vi "Read BM Messages.vi"(0 "Bus Config Info":T1, 11 "error in (no error)":errorcluster) -> (4 "VP BM Messages Read":T3[](array[typedef]) {"Data Word array" format="%x"}, 8 "Data Available":bool, 15 "error out":errorcluster)   [LabVIEW 2013, in "AIT 1553 Custom Device.lvlib"]
uses:
  AIT 1553 Custom Device.lvlib
  RT Controls/VP_BM Message.ctl
  RT Controls/AIT 1553 - Board Config Info.ctl
  RT Controls/AIT 1553 - Hardware Type.ctl
  <instrlib>/AIT 1553/AIT 1553.lvlib
  <userlib>/MIL-STD-1553/Owl1553.lvlib
  <vilib>/NI Veristand/Custom Device Tools/Custom Device Utility Library/Custom Device Utility Library.lvlib
  <vilib>/NI Veristand/Custom Device Tools/Custom Device Utility Library/RT Debug String Color Spec.ctl
panel:
  out "BM Read Exec Time":u32
  out "words read out":i32
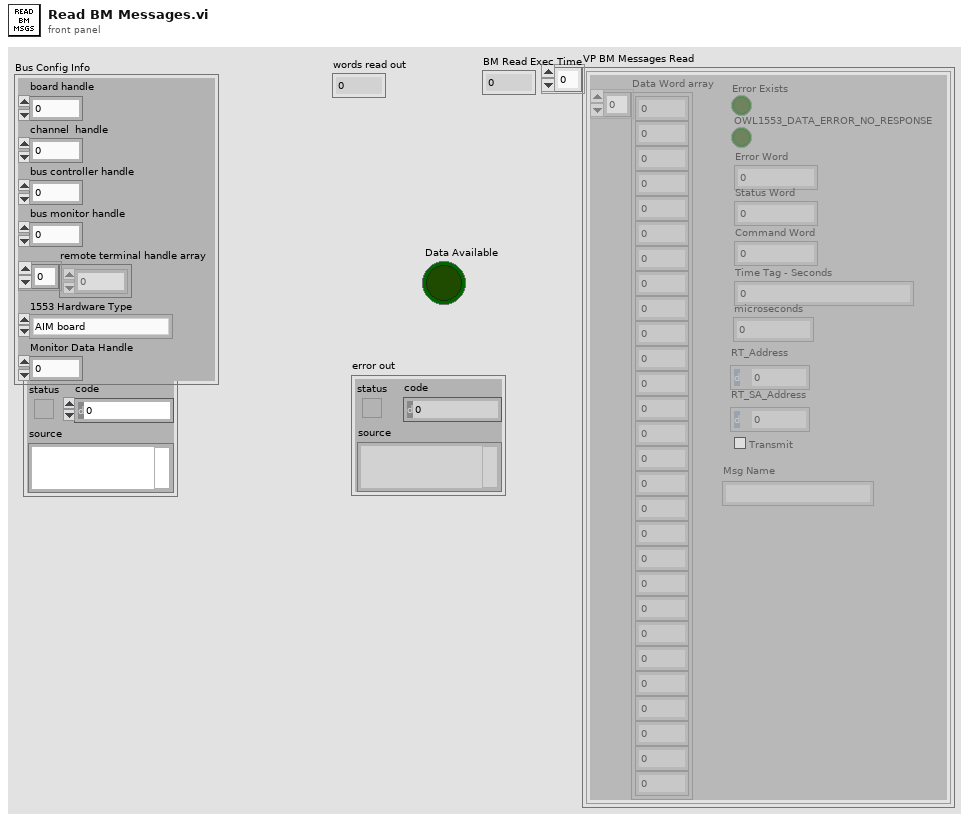
[diagram p1: front panel]
types:
  T1 = typedef "AIT 1553 Custom Device.lvlib/AIT 1553 - Board Config Info.ctl" = cluster{"board handle":u32, "channel  handle":u32, "bus controller handle":u32, "bus monitor handle":u32, "remote terminal handle array":u32[], "1553 Hardware Type":T2, "Monitor Data Handle":u32}
  T2 = typedef "AIT 1553 Custom Device.lvlib/AIT 1553 - Hardware Type.ctl" = enum16{"AIM board", "AIT Board"}
  T3 = typedef "AIT 1553 Custom Device.lvlib/VP_BM Message.ctl" = cluster{"Data Word array":u16[], "Error Exists":bool, "OWL1553_DATA_ERROR_NO_RESPONSE":bool, "Error Word":u32, "Status Word":u16, "Command Word":u16, "Time Tag - Seconds":u32, "microseconds":u32, "RT_Address":u8, "RT_SA_Address":u8, "Transmit":bool, "Msg Name":string}
  T4 = typedef "Custom Device Utility Library.lvlib/RT Debug String Color Spec.ctl" = u16
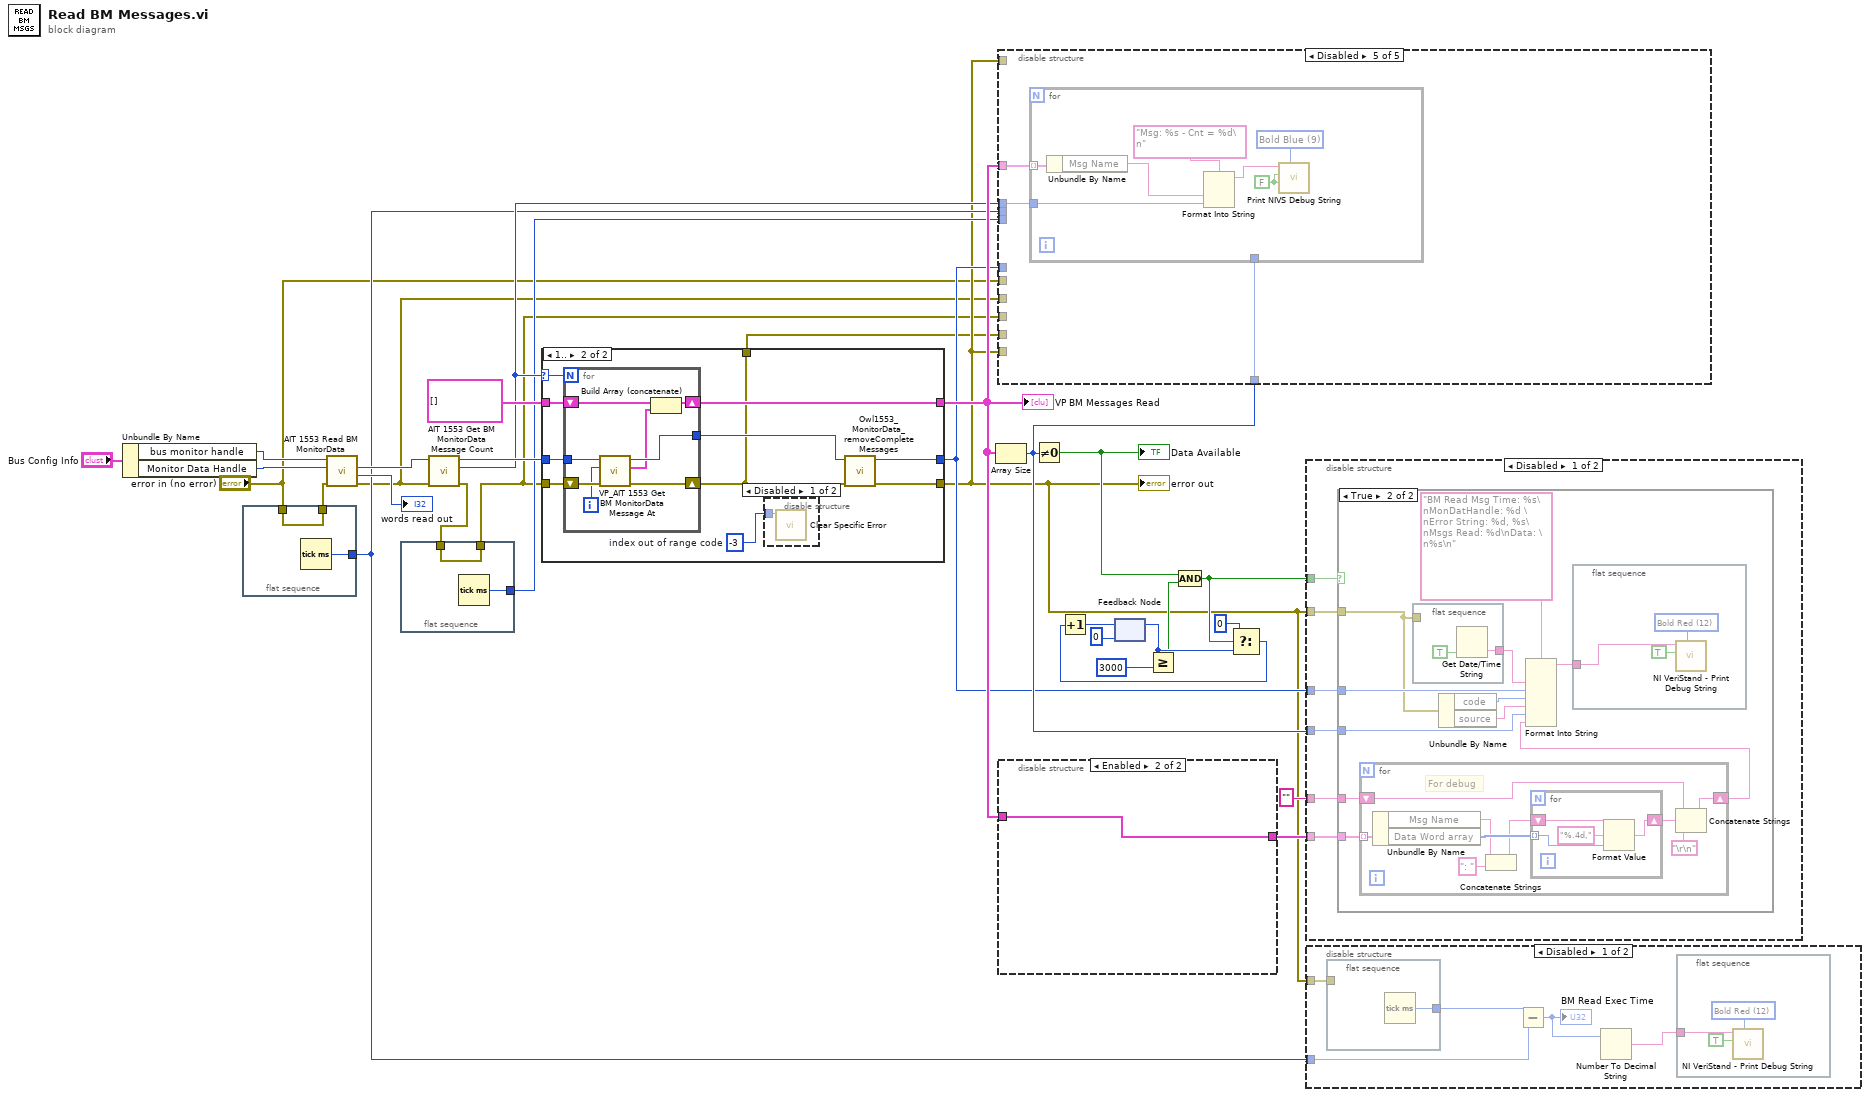
[diagram p0: block diagram]
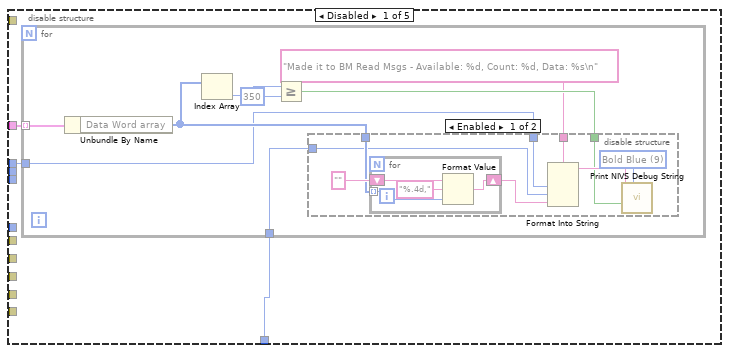
[diagram p2: hidden frame]
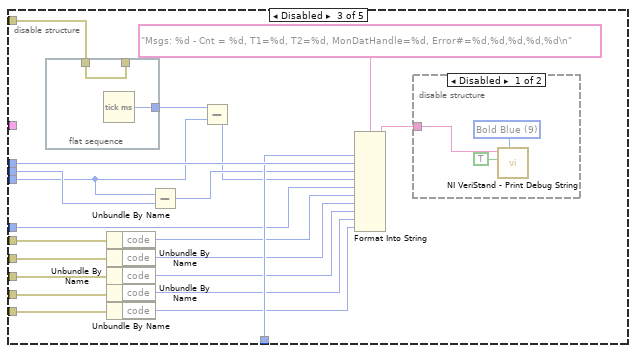
[diagram p5: hidden frame]
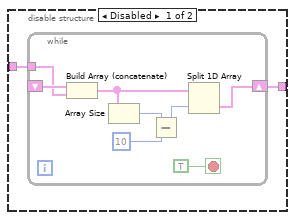
[diagram p11: hidden frame]
diagram:
  n1 = Unbundle By Name("Bus Config Info") -> ("bus monitor handle"=w5:u32, "Monitor Data Handle"=w26:u32)
  n2 = flat-sequence {
    tunnel: "error in (no error)" -> [w33]
    tunnel: [w33] -> w15
    tunnel: [w32] -> w9
    frame #0 {
      n3 = Tick Count (ms)() -> (millisecond timer value=w32:u32)
    }
  }
  n4 = call <instrlib>:"AIT 1553 Read BM MonitorData.vi"("error in"=w15, "monitor data handle in"=w26, "bus monitor handle in"=w5) -> ("error out"=w3:errorcluster, "words read out"=→"words read out":i32, "monitor data handle out"=w30:u32)  [unwired: 5 in, 1 out]
  n5 = flat-sequence {
    tunnel: w10 -> [w35]
    tunnel: [w35] -> w2
    tunnel: [w34] -> w8
    frame #0 {
      n6 = Tick Count (ms)() -> (millisecond timer value=w34:u32)
    }
  }
  n7 = call <instrlib>:"AIT 1553 Get BM MonitorData Message Count.vi"("error in"=w3, "monitor data handle in"=w30) -> ("error out"=w10:errorcluster, "message count out"=w12:u32, "monitor data handle out"=w29:u32)  [unwired: 7 in]
  n8 = case shown="1.." w12 {
    selector: w12 -> [_ w44]
    tunnel: w2 -> [w36 w48]
    tunnel: w29 -> [w37 w47]
    tunnel: T3[] [] -> [w38 w46]
    tunnel: [w38 w45] -> w14
    tunnel: [w36 w40] -> w6
    tunnel: [w37 w43] -> w7
    tunnel: [_ w39] -> w1
    frame 0, Default {
    }
    frame 1.. {
      w41 = -3  # index out of range code
      n9 = for {
        N: w44 -> [_]
        tunnel: w47 -> [w55]
        shift-right: [w52] -> w45
        shift-left: w46 -> [w53]
        tunnel: [w51] -> w42
        shift-right: [w56] -> w39
        shift-left: w48 -> [w57]
        i -> [w54]
        n10 = call "VP_AIT 1553 Get BM MonitorData Message At.vi"("error in"=w57, "message index in"=w54, "monitor data handle in"=w55) -> ("error out"=w56:errorcluster, "VP BM Message"=w50:T3[], "monitor data handle out"=w51:u32)  [unwired: 5 in]
        n11 = Build Array (concatenate)(w53, w50) -> (w52:T3[])
      }
      n12 = disable-structure shown="Disabled" {
        disable-tunnel: w41 -> [w49 _]
        frame Disabled {
          n13 = call "Clear Specific Error.vi"("code"=w49) -> ()  [unwired: 9 in, 2 out]
        }
        frame Enabled {
        }
      }
      n14 = call <userlib>:"Owl1553_MonitorData_removeCompleteMessages.vi"("error in (no error)"=w39, "monitor data handle"=w42) -> ("error out"=w40:errorcluster, "monitor data handle"=w43:u32)  [unwired: 8 in]
    }
  }
  "error out" <- w6
  "VP BM Messages Read" <- w14
  n15 = Array Size(array=w14) -> (size(s)=w13:i32)
  n16 = disable-structure shown="Disabled" {
    disable-tunnel: w14 -> [w60 _ _ _ w110]
    disable-tunnel: w13 -> [w59 _ w99 _ w109]
    disable-tunnel: w12 -> [w58 _ w102 _ w108]
    disable-tunnel: w9 -> [_ _ w97 _ _]
    disable-tunnel: w8 -> [_ _ w94 _ _]
    disable-tunnel: w6 -> [_ _ w98 _ _]
    disable-tunnel: w7 -> [_ _ w92 _ _]
    disable-tunnel: w6 -> [_ _ w88 _ _]
    disable-tunnel: "error in (no error)" -> [_ _ w91 _ _]
    disable-tunnel: w3 -> [_ _ w90 _ _]
    disable-tunnel: w2 -> [_ _ w89 _ _]
    disable-tunnel: w1 -> [_ _ w87 _ _]
    frame Disabled {
      n17 = for {
        tunnel: w60 -> [w65] mode=indexing
        tunnel: w59 -> [w62]
        tunnel: w58 -> [w61]
        n18 = Unbundle By Name(w65) -> ("Data Word array"=w68:u16[])
        n19 = Index Array(array=w68) -> (element=w67:u16)  [unwired: 1 in]
        n20 = Greater Or Equal?(x=w67, y=u16 350) -> (x >= y?=w64:bool)
        n21 = disable-structure shown="Enabled" {
          disable-tunnel: "Made it to BM Read Msgs - Available: %d, Count: %d, Data: %s\n" ("format string") -> [w76 _]
          disable-tunnel: w68 -> [w73 _]
          disable-tunnel: w64 -> [w71 _]
          disable-tunnel: w62 -> [w70 _]
          disable-tunnel: w61 -> [w69 _]
          frame Enabled {
            w72 = u16 9 items=["Plain White"=7, "Bold White"=15, "Bold Blue"=9, "Bold Green"=10, "Bold Red"=12] ("Color (Plain White)")
            n22 = for {
              tunnel: w73 -> [w78] mode=indexing
              shift-right: [w79] -> w75
              shift-left: "" ("format string") -> [w80]
              n23 = Format Value(string ("")=w80, format string="%.4d,", value (0)=w78) -> (output string=w79:string)
            }
            n24 = Format Into String(format string=w76, w69, w70, w75) -> (resulting string=w74:string)  [unwired: 2 in, 1 out]
            n25 = call "Print NIVS Debug String.vi"("Color (Plain White)"=w72, "Add to NIVS Log FIle? (T)"=w71, "Debug String"=w74) -> ()  [unwired: 7 in, 1 out]
          }
          frame Disabled {
          }
        }
      }
    }
    frame Disabled {
    }
    frame Disabled {
      n26 = flat-sequence {
        tunnel: w98 -> [w107]
        tunnel: [w107] -> _
        tunnel: [w106] -> w95
        frame #0 {
          n27 = Tick Count (ms)() -> (millisecond timer value=w106:u32)
        }
      }
      n28 = Unbundle By Name(w91) -> ("code"=w86:i32)
      n29 = Unbundle By Name(w90) -> ("code"=w85:i32)
      n30 = Unbundle By Name(w89) -> ("code"=w84:i32)
      n31 = Unbundle By Name(w87) -> ("code"=w83:i32)
      n32 = Unbundle By Name(w88) -> ("code"=w82:i32)
      n33 = Subtract(x=w94, y=w97) -> (x-y=w96:u32)
      n34 = Subtract(x=w95, y=w94) -> (x-y=w93:u32)
      n35 = Format Into String(format string="Msgs: %d - Cnt = %d, T1=%d, T2=%d, MonDatHandle=%d, Error#=%d,%d,%d,%d,%d\n", w99, w102, w96, w93, w92, w86, w85, w84, w83, w82) -> (resulting string=w101:string)  [unwired: 2 in, 1 out]
      n36 = disable-structure shown="Disabled" {
        disable-tunnel: w101 -> [w103 _]
        frame Disabled {
          w104 = T4 9 items=["Plain White"=7, "Bold White"=15, "Bold Blue"=9, "Bold Green"=10, "Bold Red"=12] ("Attribute")
          n37 = call <vilib>:"NI VeriStand - Print Debug String.vi"("Attribute"=w104, "Add to log file? (T)"=TRUE, "Message"=w103) -> ()  [unwired: 8 in, 1 out]
        }
        frame Enabled {
        }
      }
    }
    frame Enabled {
    }
    frame Disabled {
      n38 = for {
        tunnel: w110 -> [w113] mode=indexing
        tunnel: w109 -> [_]
        tunnel: w108 -> [w111]
        w114 = FALSE ("Add to NIVS Log FIle? (T)")
        w115 = u16 9 items=["Plain White"=7, "Bold White"=15, "Bold Blue"=9, "Bold Green"=10, "Bold Red"=12] ("Color (Plain White)")
        n39 = Unbundle By Name(w113) -> ("Msg Name"=w112:string)
        n40 = Format Into String(format string="Msg: %s - Cnt = %d\n", w112, w111) -> (resulting string=w117:string)  [unwired: 2 in, 1 out]
        n41 = call "Print NIVS Debug String.vi"("Color (Plain White)"=w115, "Add to NIVS Log FIle? (T)"=w114, "Append EOL? (T)"=w114, "Debug String"=w117) -> ()  [unwired: 6 in, 1 out]
      }
    }
  }
  n42 = disable-structure shown="Enabled" {
    disable-tunnel: w14 -> [w119 w128]
    disable-tunnel: [w118 w128] -> w17
    frame Disabled {
      n43 = while {
        shift-right: [w124] -> w118
        shift-left: _ -> [w126]
        tunnel: w119 -> [w125]
        stop <- TRUE stop-if-true
        n44 = Build Array (concatenate)(w126, w125) -> (w123:T3[])
        n45 = Array Size(array=w123) -> (size(s)=w122:i32)
        n46 = Subtract(x=w122, y=10 ("index")) -> (x-y=w120:i32)
        n47 = Split 1D Array(array=w123, index=w120) -> (second subarray=w124:T3[])  [unwired: 1 out]
      }
    }
    frame Enabled {
    }
  }
  n48 = Not Equal To 0?(x=w13) -> (x != 0?=w21:bool)
  "Data Available" <- w21
  n49 = feedback #1(0) -> (w19:i32)
  n50 = Greater Or Equal?(x=w19, y=3000) -> (x >= y?=w11:bool)
  n51 = Compound Arithmetic op=AND(w21, w11) -> (w16:bool)
  n52 = Select(t=0, s=w16, f=w19) -> (s? t:f=w18:i32)
  n53 = Increment(x=w18) -> (x+1=w24:i32)
  n54 = feedback-in #1(w24) -> ()
  n55 = disable-structure shown="Disabled" {
    disable-tunnel: w13 -> [w134 _]
    disable-tunnel: w6 -> [w133 _]
    disable-tunnel: w7 -> [w132 _]
    disable-tunnel: "" ("format string") -> [w131 _]
    disable-tunnel: w17 -> [w130 _]
    disable-tunnel: w16 -> [w129 _]
    frame Disabled {
      n56 = case shown="True" w129 {
        tunnel: w132 -> [_ w140]
        tunnel: w134 -> [_ w139]
        tunnel: w133 -> [_ w138]
        tunnel: w130 -> [_ w137]
        tunnel: w131 -> [_ w136]
        frame False {
        }
        frame True {
          n57 = for {
            tunnel: w137 -> [w154] mode=indexing
            shift-right: [w150] -> w135
            shift-left: w136 -> [w149]
            # "For debug"
            n58 = Unbundle By Name(w154) -> ("Msg Name"=w148:string, "Data Word array"=w153:u16[])
            n59 = Concatenate Strings(w148, ": " ("string")) -> (w146:string)
            n60 = for {
              tunnel: w153 -> [w155] mode=indexing
              shift-right: [w156] -> w152
              shift-left: w146 -> [w157]
              n61 = Format Value(string ("")=w157, format string="%.4d,", value (0)=w155) -> (output string=w156:string)
            }
            n62 = Concatenate Strings(w149, w152, "\r\n") -> (w150:string)
          }
          n63 = flat-sequence {
            tunnel: [w160] -> w141
            tunnel: w138 -> [_]
            frame #0 {
              n64 = Get Date/Time String(want seconds? (F)=TRUE) -> (time string=w160:string)  [unwired: 2 in, 1 out]
            }
          }
          n65 = Unbundle By Name(w138) -> ("code"=w144:i32, "source"=w145:string)
          n66 = Format Into String(format string="BM Read Msg Time: %s\nMonDatHandle: %d \nError String: %d, %s\nMsgs Read: %d\nData: \n%s\n", w141, w140, w144, w145, w139, w135) -> (resulting string=w143:string)  [unwired: 2 in, 1 out]
          n67 = flat-sequence {
            tunnel: w143 -> [w161]
            frame #0 {
              w163 = T4 12 items=["Plain White"=7, "Bold White"=15, "Bold Blue"=9, "Bold Green"=10, "Bold Red"=12] ("Attribute")
              n68 = call <vilib>:"NI VeriStand - Print Debug String.vi"("Attribute"=w163, "Add to log file? (T)"=TRUE, "Message"=w161) -> ()  [unwired: 8 in, 1 out]
            }
          }
        }
      }
    }
    frame Enabled {
    }
  }
  n69 = disable-structure shown="Disabled" {
    disable-tunnel: w6 -> [w168 _]
    disable-tunnel: w9 -> [w166 _]
    frame Disabled {
      n70 = flat-sequence {
        tunnel: w168 -> [_]
        tunnel: [w172] -> w167
        frame #0 {
          n71 = Tick Count (ms)() -> (millisecond timer value=w172:u32)
        }
      }
      n72 = Subtract(x=w167, y=w166) -> (x-y=w165:u32)
      "BM Read Exec Time" <- w165
      n73 = Number To Decimal String(number=w165) -> (decimal integer string=w164:string)  [unwired: 1 in]
      n74 = flat-sequence {
        tunnel: w164 -> [w169]
        frame #0 {
          w171 = T4 12 items=["Plain White"=7, "Bold White"=15, "Bold Blue"=9, "Bold Green"=10, "Bold Red"=12] ("Attribute")
          n75 = call <vilib>:"NI VeriStand - Print Debug String.vi"("Attribute"=w171, "Add to log file? (T)"=TRUE, "Message"=w169) -> ()  [unwired: 8 in, 1 out]
        }
      }
    }
    frame Enabled {
    }
  }
